vi "Create CALL msg.vi"(8 "error in":errorcluster, 10 "Call Request":T1, 11 "Request ID":u64) -> (0 "error out":errorcluster, 3 "WAMP Message":string)   [LabVIEW 2020, in "wamplv.lvlib" / "WAMP Client.lvclass"]
uses:
  WAMP Client.lvclass
  TypeDef/CALL Request Data.ctl
  API/TypeDefs/RESULT payload.ctl
  API/TypeDefs/Combined error.ctl
  API/TypeDefs/WAMP error.ctl
  TypeDef/WAMP Message Codes.ctl
  WAMP Client.lvclass/WAMP Client.ctl
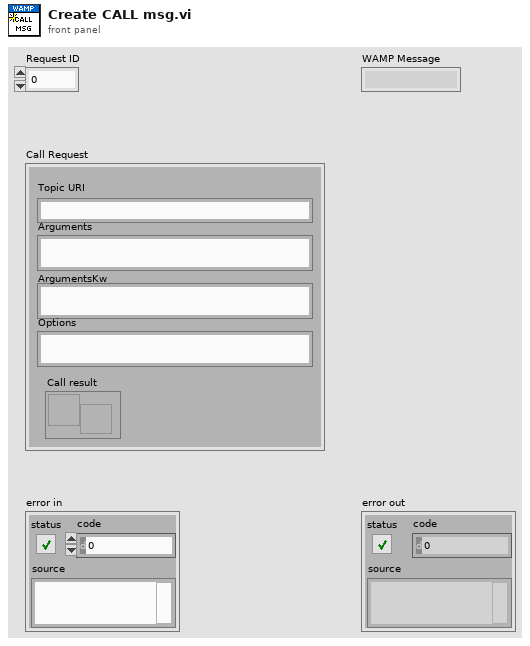
[diagram p1: front panel]
types:
  T1 = typedef "wamplv.lvlib/WAMP Client.lvclass/CALL Request Data.ctl" = cluster{"Topic URI":string, "Arguments":string, "ArgumentsKw":string, "Options":string, "Call result":refnum<notifier>}
  T2 = typedef "wamplv.lvlib/WAMP Client.lvclass/WAMP Message Codes.ctl" = u16
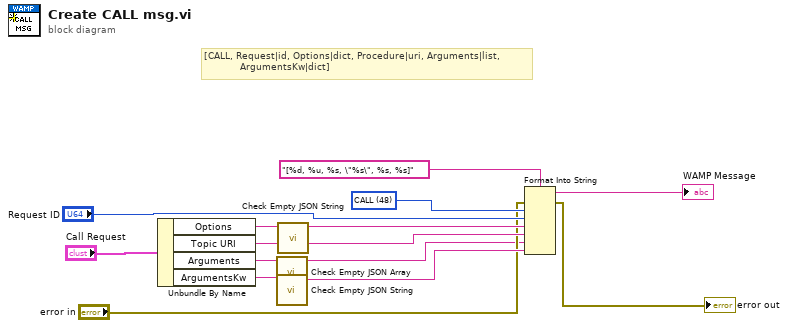
[diagram p0: block diagram]
diagram:
  w7 = T2 48 items=["HELLO"=1, "WELCOME"=2, "ABORT"=3, "GOODBYE"=6, "ERROR"=8, "PUBLISH"=16, "PUBLISHED"=17, "SUBSCRIBE"=32, "SUBSCRIBED"=33, "UNSUBSCRIBE"=34, "UNSUBSCRIBED"=35, "EVENT"=36, "CALL"=48, "RESULT"=59, "REGISTER"=64, "REGISTERED"=65, "UNREGISTER"=66, "UNREGISTERED"=67, "INVOCATION"=68, "YIELD"=70] ("Message Codes")
  # "[CALL, Request|id, Options|dict, Procedure|uri, Arguments|list,\n            ArgumentsKw|dict]"
  n1 = Unbundle By Name("Call Request") -> ("Options"=w12:string, "Topic URI"=w8:string, "Arguments"=w2:string, "ArgumentsKw"=w10:string)
  n2 = call "Check Empty JSON Array.vi"("JSON in"=w2) -> ("JSON out"=w1:string)  [unwired: 10 in]
  n3 = call "Check Empty JSON String.vi"("JSON in"=w10) -> ("JSON out"=w11:string)  [unwired: 10 in]
  n4 = call "Check Empty JSON String.vi"("JSON in"=w12) -> ("JSON out"=w13:string)  [unwired: 10 in]
  n5 = Format Into String(format string="[%d, %u, %s, \"%s\", %s, %s]" ("element"), error in="error in", w7, "Request ID", w13, w8, w1, w11) -> (resulting string=→"WAMP Message":string, error out=→"error out":errorcluster)  [unwired: 1 in]
